vi "File Unicode To ANSCII.vi"(0 "file in":path) -> (14 "file out":path)   [LabVIEW 2013]
panel:
  out "unicode-bigendian":bool
  out "unicode":bool
  out "output string":string
  out "error out":errorcluster
  in  "error in":errorcluster
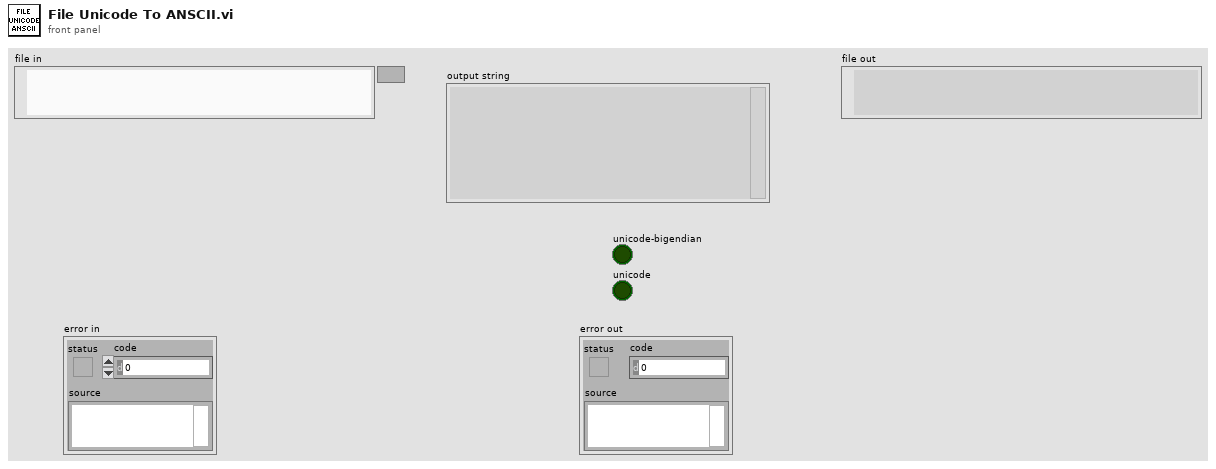
[diagram p1: front panel]
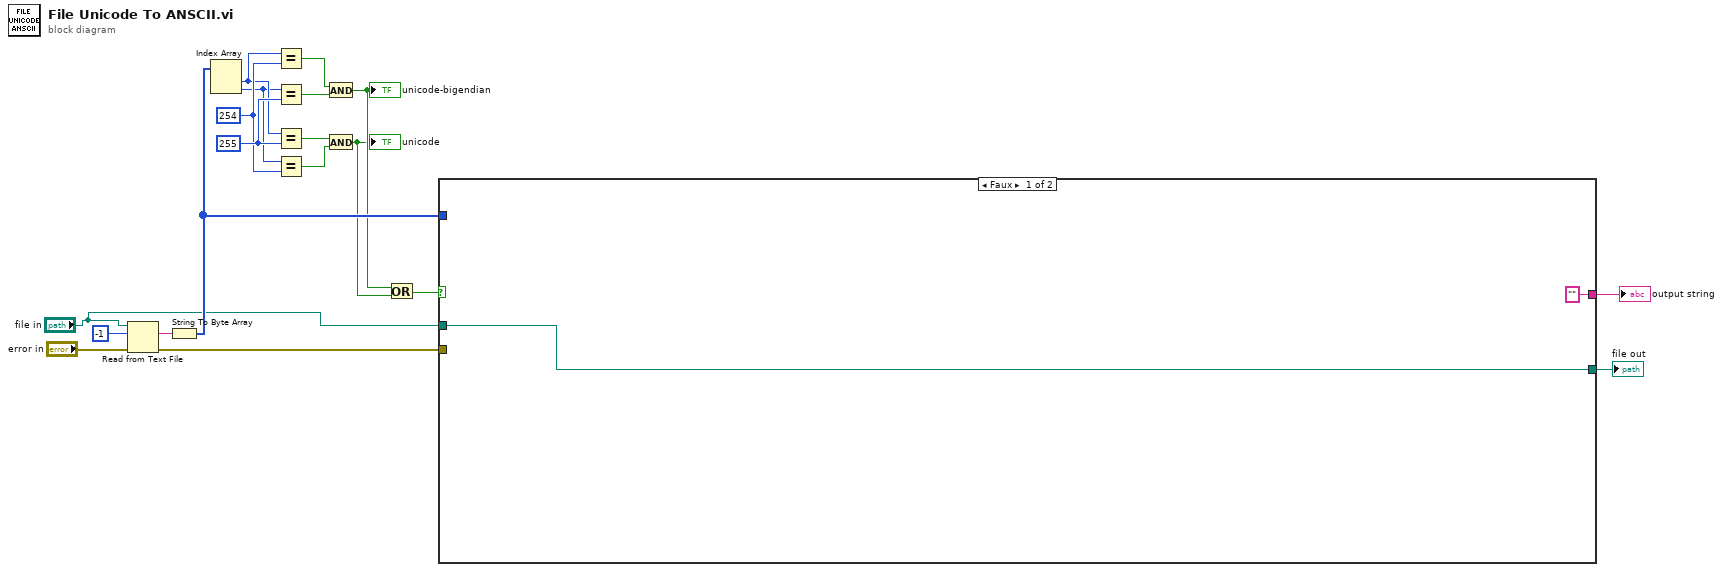
[diagram p0: block diagram]
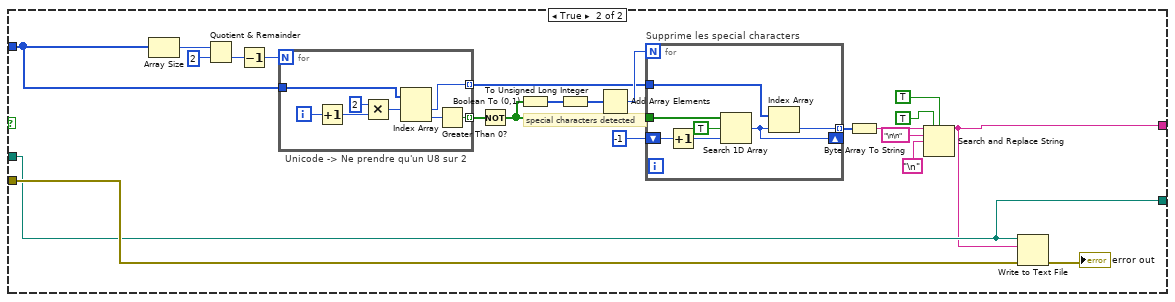
[diagram p2: hidden frame]
diagram:
  w18 = u8 254 ("y")
  w19 = u8 255 ("y")
  n1 = Read from Text File(file (use dialog)="file in", count=-1 ("nombre"), error in="error in") -> (text=w8:string, error out=w7:errorcluster)  [unwired: 1 in, 2 out]
  n2 = String To Byte Array(string=w8) -> (unsigned byte array=w13:u8[])
  n3 = Index Array(array=w13) -> (element #1=w12:u8, element #2=w11:u8)  [unwired: 2 in]
  n4 = Equal?(x=w12, y=w18) -> (x = y?=w16:bool)
  n5 = Equal?(x=w11, y=w19) -> (x = y?=w17:bool)
  n6 = Equal?(x=w12, y=w19) -> (x = y?=w15:bool)
  n7 = Equal?(x=w11, y=w18) -> (x = y?=w14:bool)
  n8 = And(x=w16, y=w17) -> (x .and. y?=w5:bool)
  "unicode-bigendian" <- w5
  n9 = And(x=w15, y=w14) -> (x .and. y?=w4:bool)
  "unicode" <- w4
  n10 = Or(x=w5, y=w4) -> (x .or. y?=w3:bool)
  n11 = case shown="Faux" w3 {
    tunnel: w13 -> [_ w41]
    tunnel: w7 -> [_ w25]
    tunnel: "file in" -> [w21 w23]
    tunnel: [w21 w23] -> w2
    tunnel: ["" ("result string") w22] -> w1
    frame False {
    }
    frame True {
      # "special characters detected"
      n12 = Array Size(array=w41) -> (size(s)=w43:i32)
      n13 = Quotient & Remainder(x=w43, y=2) -> (floor(x/y)=w40:i32)  [unwired: 1 out]
      n14 = Decrement(x=w40) -> (x-1=w39:i32)
      n15 = for "Unicode -> Ne prendre qu'un U8 sur 2" {
        N: w39 -> [_]
        tunnel: w41 -> [w50]
        tunnel: [w47] -> w30 mode=indexing
        tunnel: [w44] -> w32 mode=indexing
        i -> [w46]
        n16 = Increment(x=w46) -> (x+1=w45:i32)
        n17 = Multiply(x=2, y=w45) -> (x*y=w49:i32)
        n18 = Index Array(array=w50, index #1=w49) -> (element #1=w47:u8, element #2=w48:u8)  [unwired: 1 in]
        n19 = Greater Than 0?(x=w48) -> (x > 0?=w44:bool)
      }
      n20 = Not(x=w32) -> (.not. x?=w29:bool[])
      n21 = Boolean To (0,1)(Boolean=w29) -> (0, 1=w34:i16[])
      n22 = To Unsigned Long Integer(number=w34) -> (unsigned 32bit integer=w33:u32[])
      n23 = Add Array Elements(numeric array=w33) -> (sum=w35:u32)
      n24 = for "Supprime les special characters" {
        N: w35 -> [_]
        tunnel: w30 -> [w52]
        tunnel: w29 -> [w58]
        shift-right: [w55] -> _
        shift-left: -1 ("start index (0)") -> [w56]
        tunnel: [w54] -> w31 mode=indexing
        n25 = Increment(x=w56) -> (x+1=w53:i32)
        n26 = Search 1D Array(1D array=w58, element=TRUE, start index (0)=w53) -> (index of element=w55:i32)
        n27 = Index Array(array=w52, index=w55) -> (element=w54:u8)
      }
      n28 = Byte Array To String(unsigned byte array=w31) -> (string=w37:string)
      n29 = Search and Replace String(replace all?=TRUE ("replace all? (F)"), case sensitive?=TRUE ("ignorer la casse ? (F)"), input string=w37, search string="\n\n", replace string="\n") -> (result string=w22:string)  [unwired: 3 in, 3 out]
      n30 = Write to Text File(file (use dialog)=w23, text=w22, error in=w25) -> (error out=→"error out":errorcluster)  [unwired: 1 in, 2 out]
    }
  }
  "file out" <- w2
  "output string" <- w1
